vi "MagX List.vi"(2 "Experiments list":i32(listbox)=-1, 6 "Days range":dbl=90.0, 8 "error in":errorcluster, 9 "Current station in":string, 10 "Initial Selection":string, 11 "Hub URL":string="magx.lanl.gov") -> (0 "error out":errorcluster, 1 "OK":bool, 3 "Experiment info":T1, 5 "Online":bool)   [LabVIEW 2025]
uses:
  Experiment info.ctl
panel:
  in  "Search":string
  out "Current station":string
  out "Selection":string
  in  "Select":bool
  out "Experiments":T1[](array[typedef])
  out "resulting string":string
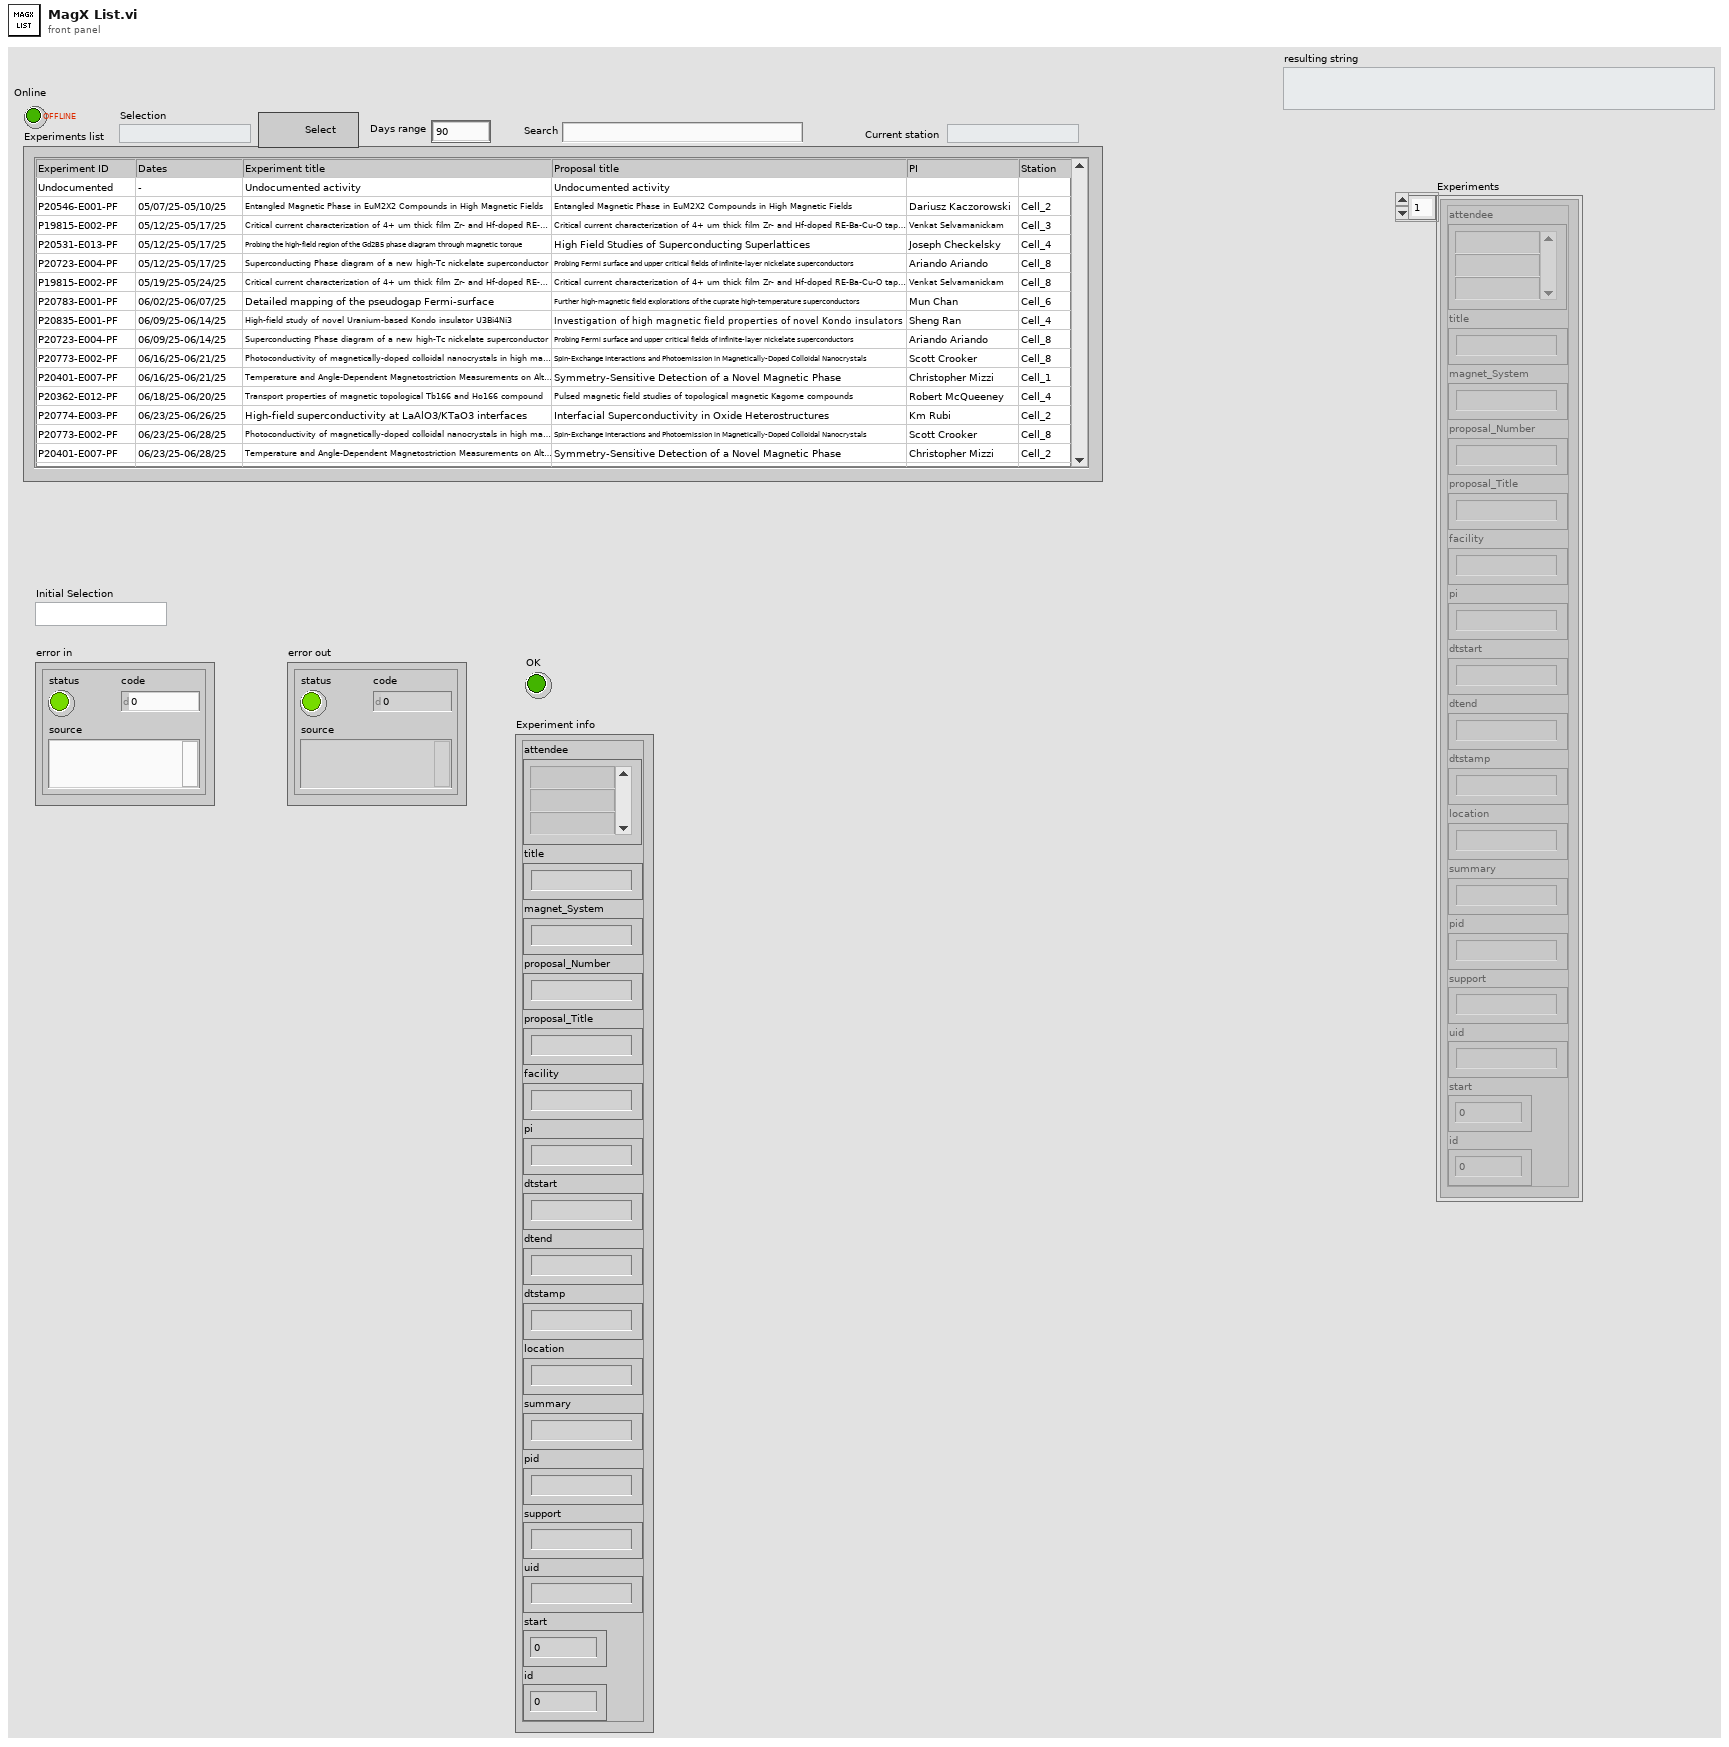
[diagram p1: front panel]
types:
  T1 = typedef "Experiment info.ctl" = cluster{"attendee":string[], "title":string, "magnet_System":string, "proposal_Number":string, "proposal_Title":string, "facility":string, "pi":string, "dtstart":string, "dtend":string, "dtstamp":string, "location":string, "summary":string, "pid":string, "support":string, "uid":string, "start":u64, "id":u64}
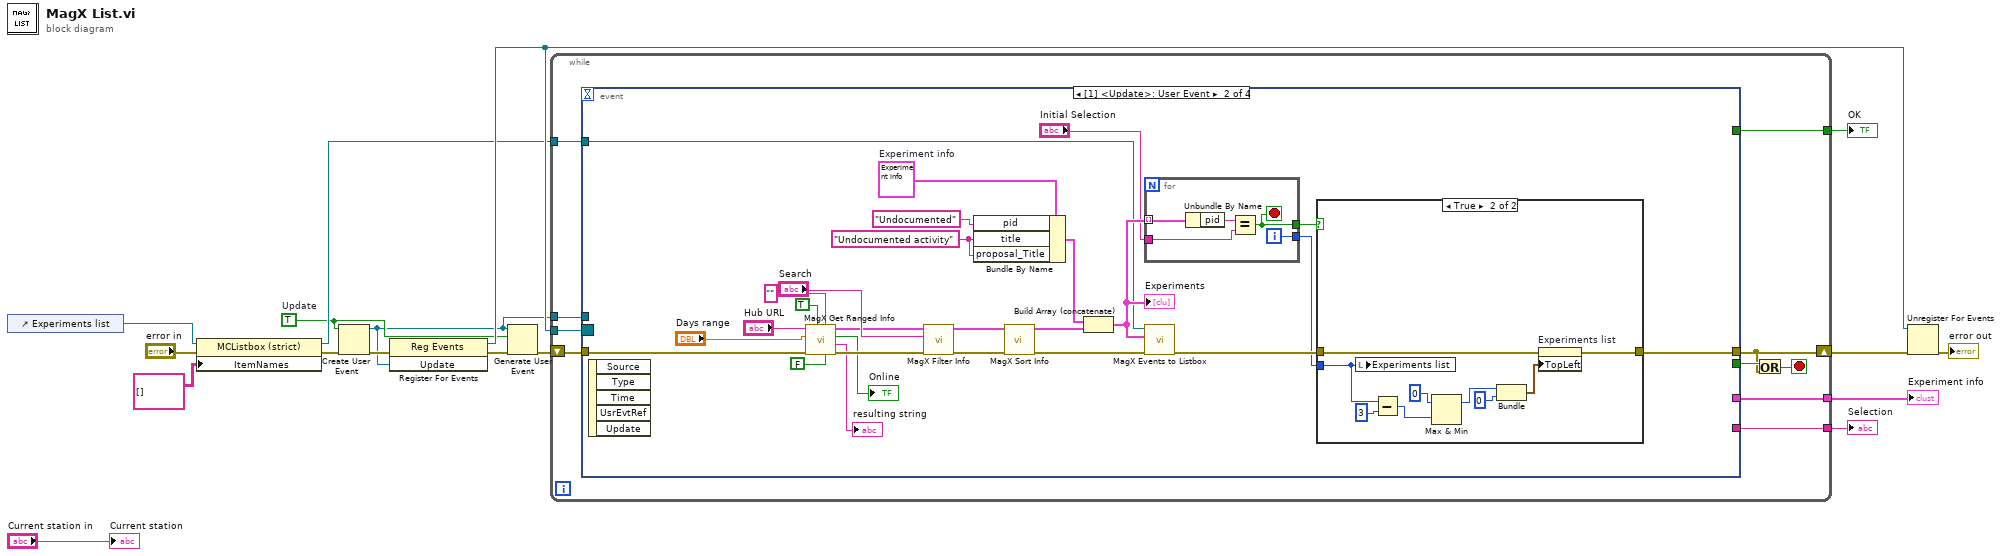
[diagram p0: block diagram]
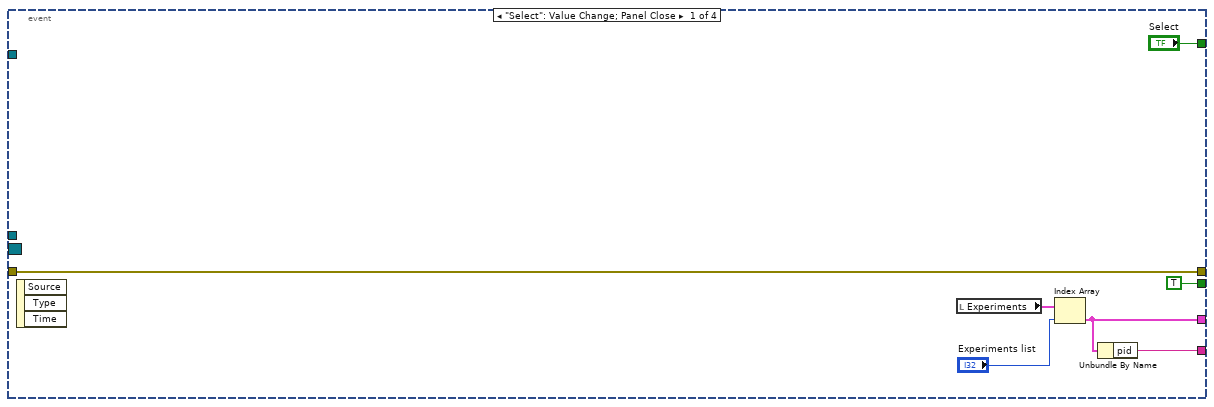
[diagram p2: hidden frame]
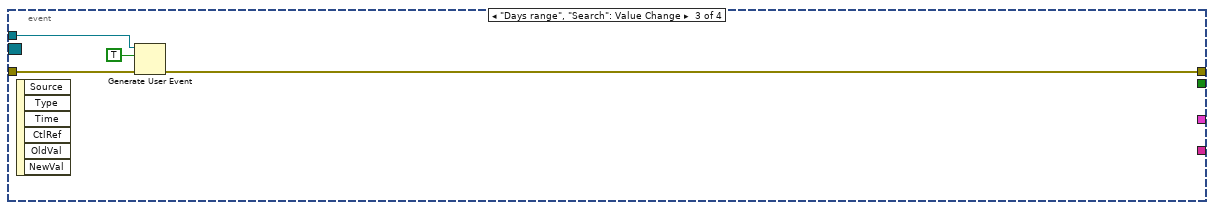
[diagram p4: hidden frame]
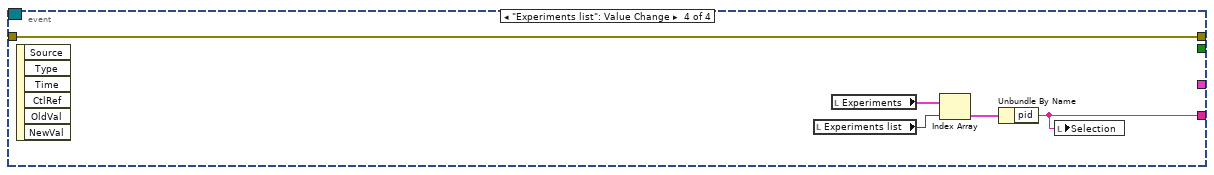
[diagram p5: hidden frame]
diagram:
  w2 = TRUE  # Update
  n1 = control-ref of="Experiments list"() -> (w9:refnum<vi>)
  n2 = property class="MCListbox (strict)"(reference=w9, error in="error in", "ItemNames"=string[][] [] ("Item Names")) -> (reference out=w8:refnum<vi>, error out=w6:errorcluster)
  n3 = Create User Event(user event datatype=w2, error in=w6) -> (user event=w1:refnum<user-event>, error out=w13:errorcluster)
  n4 = register-events(error in=w13, w1) -> (reference out=w10:refnum<event-registration>, error out=w4:errorcluster)  [unwired: 1 in]
  n5 = Generate User Event(user event=w1, event data cluster=w2, error in=w4) -> (error out=w3:errorcluster)  [unwired: 1 in, 1 out]
  n6 = while {
    shift-right: [w24] -> w12
    shift-left: w3 -> [w27]
    tunnel: [w23] -> w17
    tunnel: [w22] -> w16
    tunnel: [w21] -> w15
    tunnel: w10 -> [w20]
    tunnel: w8 -> [w19]
    tunnel: w1 -> [w18]
    stop <- w25 stop-if-true
    n7 = event shown="[1] <Update>: User Event" {
      selector: w20 -> [_ _ _ _]
      dyn-events: _ -> [_ _ _ _]
      timeout: _ -> [_ _ _ _]
      tunnel: w27 -> [w34 w44 w79 w84]
      tunnel: [w34 w49 w78 w84] -> w24
      tunnel: [TRUE ("Select") _ _ _] -> w26
      tunnel: [w31 _ _ w80] -> w23
      tunnel: [w29 _ _ _] -> w22
      tunnel: ["Select" _ _ _] -> w21
      tunnel: w19 -> [_ w48 _ _]
      tunnel: w18 -> [_ _ w77 _]
      event "Select": Value Change; Panel Close {
        n8 = event-data() -> ()  [unwired: 1 in, 3 out]
        n9 = local read "Experiments"() -> (w33:T1[])
        n10 = Index Array(array=w33, index="Experiments list") -> (element=w29:T1)
        n11 = Unbundle By Name(w29) -> ("pid"=w31:string)
      }
      event User Event {
        w50 = "Undocumented activity"
        w52 = T1 {"attendee"=[], "title"="", "magnet_System"="", "proposal_Number"="", "proposal_Title"="", "facility"="", "pi"="", "dtstart"="", "dtend"="", "dtstamp"="", "location"="", "summary"="", "pid"="", "support"="", "uid"="", "start"=0, "id"=0}  # Experiment info
        n12 = event-data() -> ()  [unwired: 1 in, 5 out]
        n13 = call "MagX Get Ranged Info.vi"("Save cache"=FALSE, "Station"="", "Use cache"=TRUE, "error in"=w44, "Days range"="Days range", "Hub URL"="Hub URL") -> ("error out"=w41:errorcluster, "resulting string"=→"resulting string":string, "Online"=→"Online":bool, "Data out"=w40:T1[])  [unwired: 2 in]
        n14 = call "MagX Filter Info.vi"("error in"=w41, "Search"="Search", "Data in"=w40) -> ("error out"=w47:errorcluster, "Data out"=w46:T1[])  [unwired: 7 in]
        n15 = Bundle By Name(cluster=w52, "pid"="Undocumented", "title"=w50, "proposal_Title"=w50) -> (w58:T1)
        n16 = call "MagX Sort Info.vi"("error in"=w47, "Data in"=w46) -> ("error out"=w59:errorcluster, "Data out"=w60:T1[])  [unwired: 8 in]
        n17 = Build Array (concatenate)(w58, w60) -> (w57:T1[])
        "Experiments" <- w57
        n18 = for {
          tunnel: w57 -> [w75] mode=indexing
          tunnel: "Initial Selection" -> [w74]
          tunnel: [w72] -> w55
          tunnel: [w71] -> w54
          i -> [w72]
          stop <- w71 stop-if-true
          n19 = Unbundle By Name(w75) -> ("pid"=w73:string)
          n20 = Equal?(x=w73, y=w74) -> (x = y?=w71:bool)
        }
        n21 = call "MagX Events to Listbox.vi"("error in"=w59, "Experiments"=w57, "Listbox ref"=w48) -> ("error out"=w56:errorcluster)  [unwired: 7 in, 1 out]
        n22 = case shown="True" w54 {
          tunnel: w55 -> [_ w70]
          tunnel: w56 -> [w61 w66]
          tunnel: [w61 w65] -> w49
          frame False {
          }
          frame True {
            n23 = local write "Experiments list"(w70) -> ()
            n24 = Subtract(x=w70, y=3) -> (x-y=w63:i32)
            n25 = Max & Min(x=0, y=w63) -> (max(x,y)=w64:i32)  [unwired: 1 out]
            n26 = Bundle(w64, 0) -> (w69:cluster{i32, i32})  [unwired: 1 in]
            n27 = property on="Experiments list" class="MCListbox (strict)"(error in=w66, "TopLeft"=w69) -> (error out=w65:errorcluster)  [unwired: 1 in, 1 out]
          }
        }
      }
      event "Days range", "Search": Value Change {
        n28 = event-data() -> ()  [unwired: 1 in, 6 out]
        n29 = Generate User Event(user event=w77, event data cluster=TRUE ("event data"), error in=w79) -> (error out=w78:errorcluster)  [unwired: 1 in, 1 out]
      }
      event "Experiments list": Value Change {
        n30 = event-data() -> ()  [unwired: 1 in, 6 out]
        n31 = local read "Experiments list"() -> (w81:i32)
        n32 = local read "Experiments"() -> (w83:T1[])
        n33 = Index Array(array=w83, index=w81) -> (element=w82:T1)
        n34 = Unbundle By Name(w82) -> ("pid"=w80:string)
        n35 = local write "Selection"(w80) -> ()
      }
    }
    n36 = Or(x=w26, y=w24) -> (x .or. y?=w25:bool)
  }
  "Selection" <- w17
  "Experiment info" <- w16
  "OK" <- w15
  n37 = Unregister For Events(event registration refnum=w10, error in=w12) -> (error out=→"error out":errorcluster)
  "Current station" <- "Current station in"
